vi "RTS Macro Extract Standard Compressor Cycles.vi"(0 "Time":dbl[](array[numeric]) format="%<%H:%M:%S>t", 5 "Power (W)":dbl[](array[numeric]), 9 "Power Factor":dbl[](array[numeric]), 11 "Error In":errorcluster) -> (3 "Average Compressor Power (Watts)":dbl format="%0.2f", 4 "Standard Compressor Cycles Times":dbl[](array[numeric]) format="%<%H:%M:%S>t", 6 "Upper 3 Sig Limit":dbl, 10 "Lower 3 Sig Limit":dbl, 15 "Error Out":errorcluster)   [LabVIEW 2016]
panel:
  out "Filtered Compressor Power Chart (No Defrost)":cluster{dbl[], dbl[]}(graph)
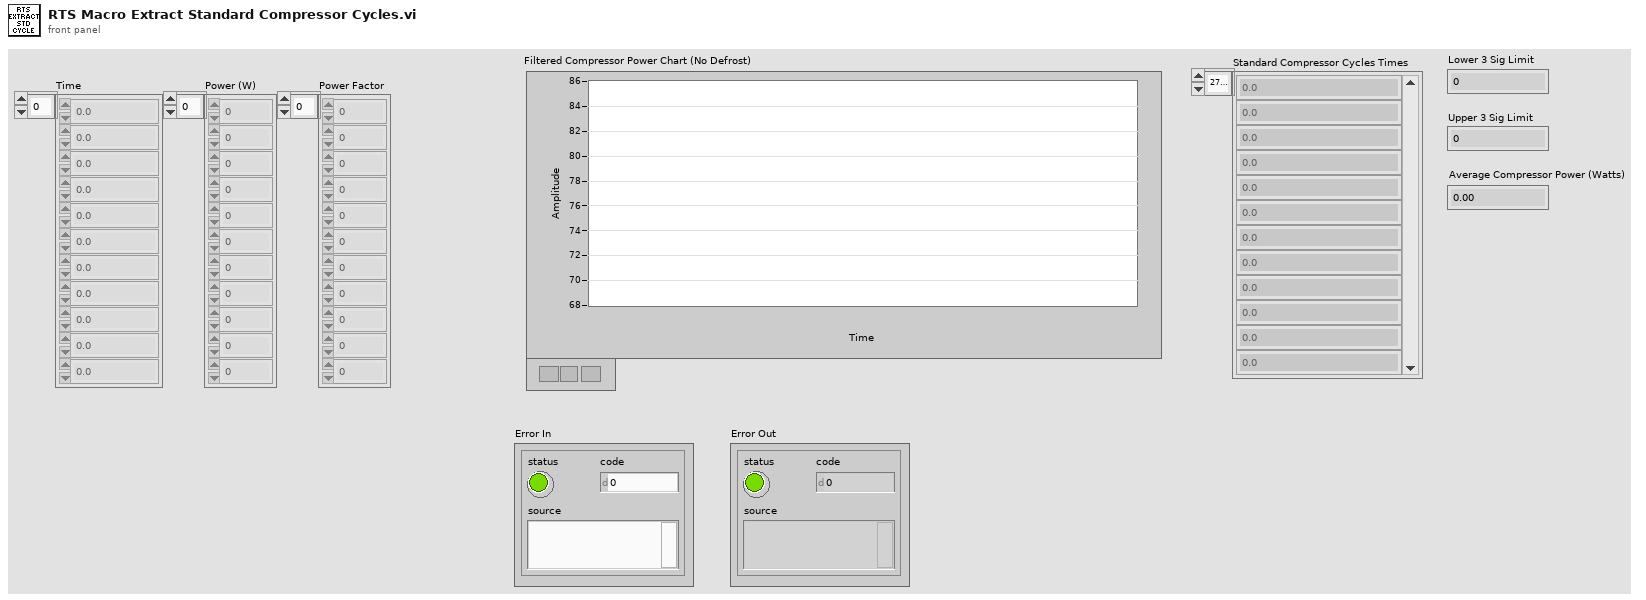
[diagram p1: front panel]
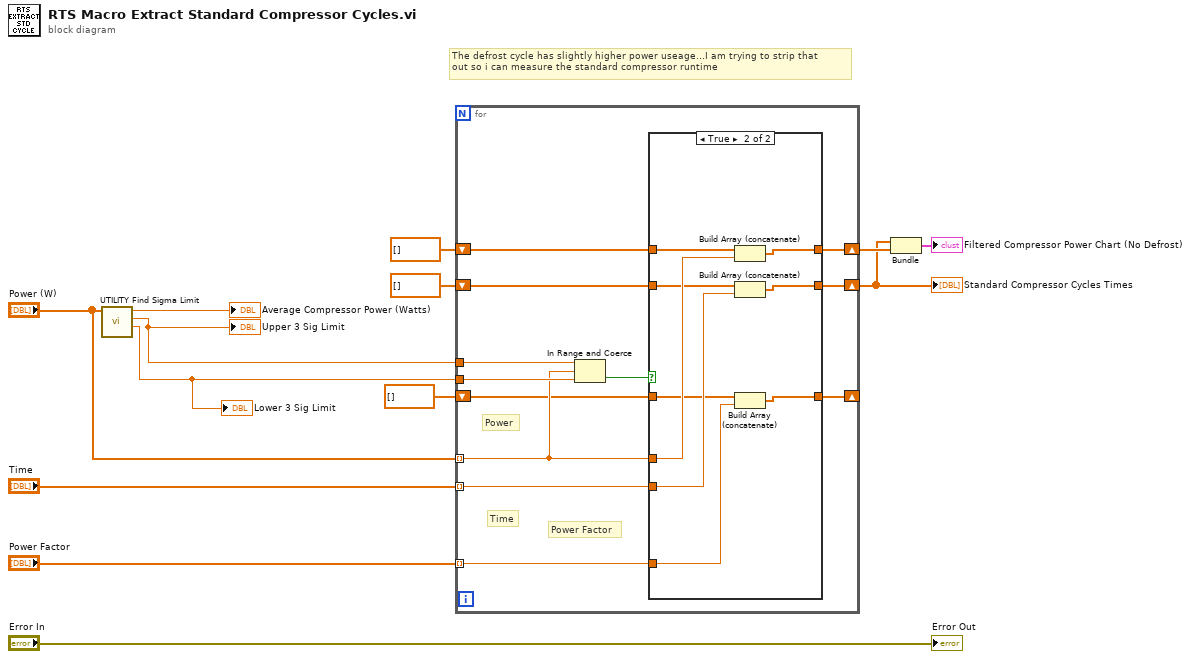
[diagram p0: block diagram]
diagram:
  # "The defrost cycle has slightly higher power useage...I am trying to strip that \nout so i can measure the standard compressor runtime"
  n1 = call "UTILITY Find Sigma Limit.vi"("Filtered Power Data (W)"="Power (W)") -> ("Lower 3 Sig Limit"=w2:dbl, "Upper 3 Sig Limit"=w1:dbl, "Average Compressor Power (Watts)"=→"Average Compressor Power (Watts)":dbl)  [unwired: 7 in, 1 out]
  "Upper 3 Sig Limit" <- w1
  "Lower 3 Sig Limit" <- w2
  n2 = for {
    tunnel: "Time" -> [w17] mode=indexing
    tunnel: "Power (W)" -> [w20] mode=indexing
    tunnel: w2 -> [w25]
    tunnel: w1 -> [w24]
    shift-right: [w22] -> w13
    shift-left: dbl[] [] -> [w23]
    shift-right: [w18] -> w4
    shift-left: dbl[] [] -> [w19]
    tunnel: "Power Factor" -> [w15] mode=indexing
    shift-right: [w14] -> _
    shift-left: dbl[] [] -> [w16]
    # "Power"
    # "Time"
    # "Power Factor"
    n3 = In Range and Coerce(upper limit=w24, x=w20, lower limit=w25) -> (In Range?=w21:bool)  [unwired: 1 out]
    n4 = case shown="True" w21 {
      tunnel: w23 -> [w28 w37]
      tunnel: [w28 w36] -> w22
      tunnel: w20 -> [_ w35]
      tunnel: w19 -> [w27 w34]
      tunnel: [w27 w33] -> w18
      tunnel: w17 -> [_ w32]
      tunnel: w16 -> [w26 w31]
      tunnel: w15 -> [_ w30]
      tunnel: [w26 w29] -> w14
      frame False {
      }
      frame True {
        n5 = Build Array (concatenate)(w37, w35) -> (w36:dbl[])
        n6 = Build Array (concatenate)(w34, w32) -> (w33:dbl[])
        n7 = Build Array (concatenate)(w31, w30) -> (w29:dbl[])
      }
    }
  }
  "Standard Compressor Cycles Times" <- w4
  n8 = Bundle(w4, w13) -> (→"Filtered Compressor Power Chart (No Defrost)":cluster{dbl[], dbl[]})  [unwired: 1 in]
  "Error Out" <- "Error In"
